vi "Binary Morphological Reconstruction.vi"() -> ()   [LabVIEW 2014]
doc: "This example demonstrates the use of binary morphological reconstruction in the particle analysis. The example allows you to keep the particles completely inside the ROI, completely outside the ROI or on the ROI."
uses:
  <vilib>/vision/NI_Vision_Development_Module.lvlib
panel:
  in  "Operation":T1(ring)
  out "Reconstructed Image":T2(plugin-control)
  out "Image":T2(plugin-control)
  in  "Stop":bool
  # "Overview: Demonstrate the use of the Binary Morphology Reconstruction feature of Vision Development Module.\nRequirements: Vision Development Module.\nInstructions:\n1. Run the VI.\n2. Select the ROI in which you want to filter the objects. Press the <Ctrl> key to select multiple ROIs. \n3. Choose the required \"Operation\".\n  - Inner particles: Keeps all the particles completely inside the ROI.\n  - Outer particles: Keeps the particles completely outside the ROI.\n  - Boundary particles: Keeps the particles which are touching the boundary."
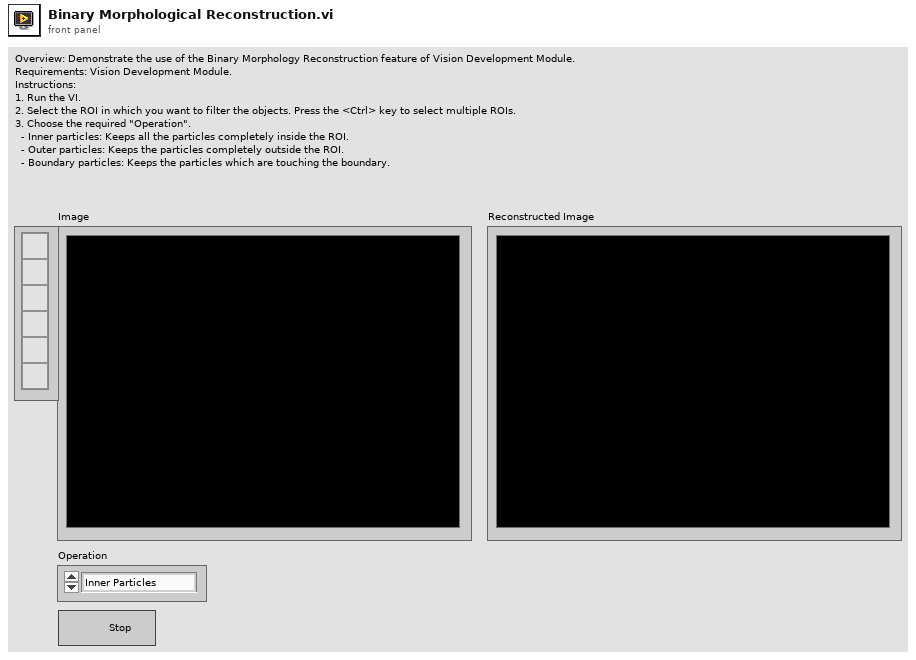
[diagram p1: front panel]
types:
  T1 = enum16{"Inner Particles", "Outer Particles", "Boundary Particles"}
  T2 = typedef "IMAQ Image.ctl" = refnum<image>
  T3 = typedef "Image Type" = u32
  T4 = cluster{"Global Rectangle":i32[], "Contours":cluster{"Contour Type":u32, "ROI Type":u32, "Points":i32[]}[]}
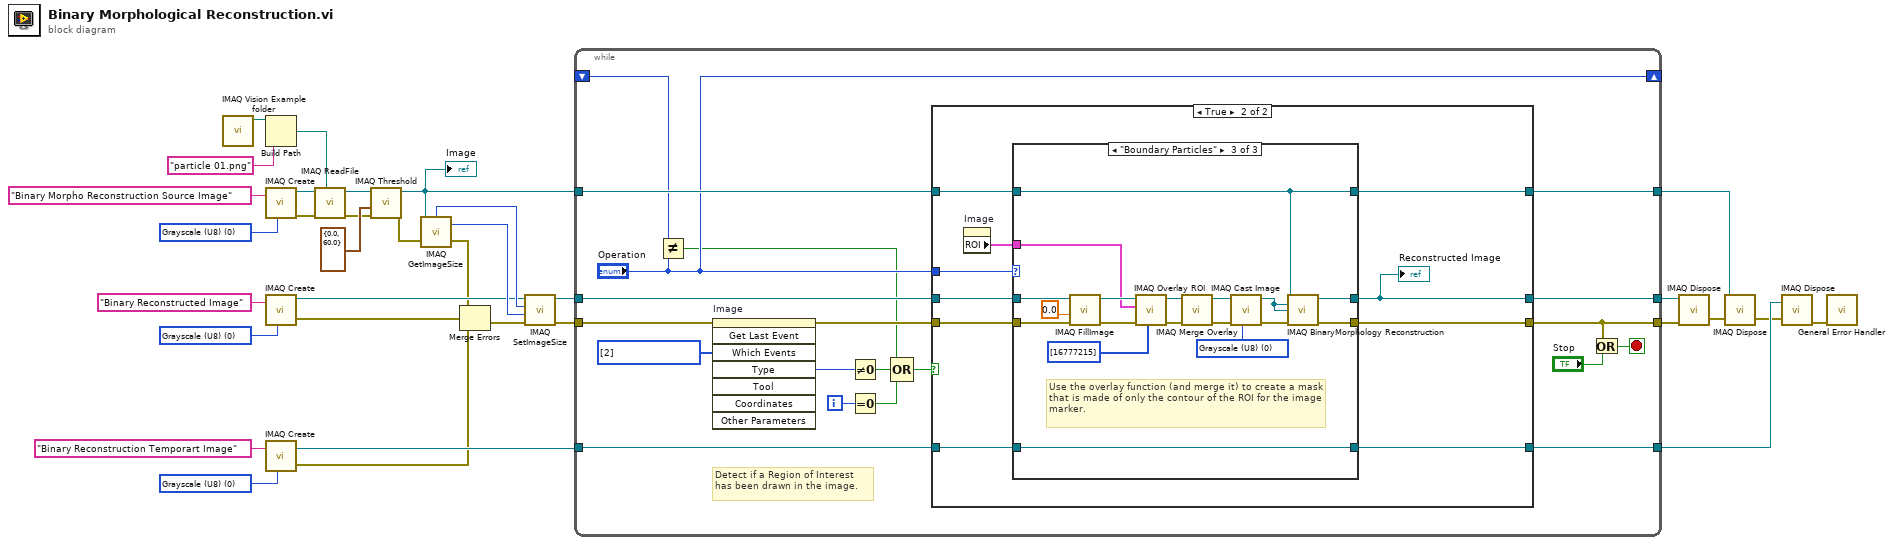
[diagram p0: block diagram]
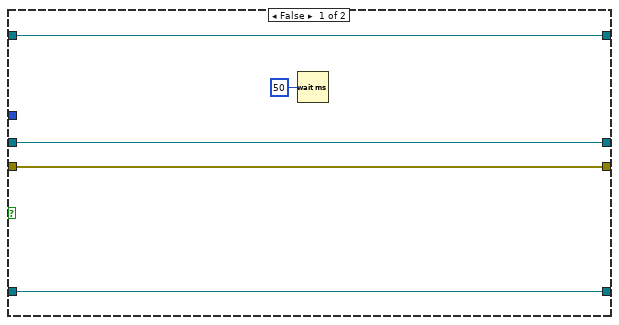
[diagram p2: hidden frame]
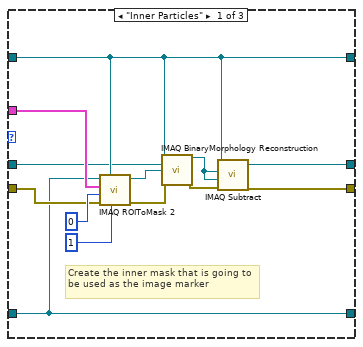
[diagram p3: hidden frame]
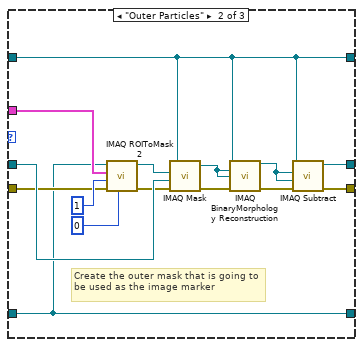
[diagram p4: hidden frame]
diagram:
  w23 = T3 0 items=["Grayscale (U8)", "Grayscale (I16)", "Grayscale (SGL)", "Complex (CSG)", "RGB (U32)", "HSL (U32)", "RGB (U64)", "Grayscale (U16)"] ("Image Type")
  w25 = T3 0 items=["Grayscale (U8)", "Grayscale (I16)", "Grayscale (SGL)", "Complex (CSG)", "RGB (U32)", "HSL (U32)", "RGB (U64)", "Grayscale (U16)"] ("Image Type")
  w26 = T3 0 items=["Grayscale (U8)", "Grayscale (I16)", "Grayscale (SGL)", "Complex (CSG)", "RGB (U32)", "HSL (U32)", "RGB (U64)", "Grayscale (U16)"] ("Image Type")
  n1 = call "IMAQ Vision Example folder.vi"() -> ("Example Image Path"=w32:path)  [unwired: 11 in]
  n2 = Build Path(base path=w32, name or relative path="particle 01.png") -> (appended path=w1:path)
  n3 = call "IMAQ Create"("Image Name"="Binary Morpho Reconstruction Source Image", "Image Type"=w25) -> ("New Image"=w29:T2, "error out"=w14:errorcluster)  [unwired: 2 in, 1 out]
  n4 = call "IMAQ Create"("Image Name"="Binary Reconstructed Image", "Image Type"=w26) -> ("New Image"=w19:T2, "error out"=w11:errorcluster)  [unwired: 2 in, 1 out]
  n5 = call "IMAQ Create"("Image Name"="Binary Reconstruction Temporart Image", "Image Type"=w23) -> ("New Image"=w20:T2, "error out"=w10:errorcluster)  [unwired: 2 in, 1 out]
  n6 = call "IMAQ ReadFile"("File Path"=w1, "error in (no error)"=w14, "Image"=w29) -> ("error out"=w13:errorcluster, "Image Out"=w17:T2)  [unwired: 2 in, 5 out]
  n7 = call "IMAQ Threshold"("error in (no error)"=w13, "Range"=cluster{"Lower value":sgl, "Upper value":sgl} {"Lower value"=0.0, "Upper value"=60.0}, "Image Src"=w17) -> ("error out"=w12:errorcluster, "Image Dst Out"=w15:T2)  [unwired: 3 in, 4 out]
  "Image" <- w15
  n8 = call "IMAQ GetImageSize"("Image"=w15, "error in (no error)"=w12) -> ("Y Resolution"=w21:i32, "X Resolution"=w22:i32, "error out"=w7:errorcluster)  [unwired: 2 out]
  n9 = Merge Errors(w7, w11, w10) -> (w9:errorcluster)
  n10 = call "IMAQ SetImageSize"("error in (no error)"=w9, "Y Resolution"=w21, "X Resolution"=w22, "Image"=w19) -> ("error out"=w8:errorcluster, "Image Out"=w18:T2)  [unwired: 1 out]
  n11 = while {
    tunnel: w15 -> [w53]
    tunnel: w18 -> [w52]
    tunnel: [w51] -> w28
    tunnel: [w50] -> w27
    tunnel: w20 -> [w49]
    shift-right: ["Operation"] -> _
    shift-left: _ -> [w48]
    tunnel: w8 -> [w44]
    tunnel: [w36] -> w5
    tunnel: [w42] -> w6
    i -> [w39]
    stop <- w34 stop-if-true
    w45 = i32[] [2] items=["No Event"=0, "Click Event"=1, "Draw Event"=2, "Size Event"=4, "Scroll Event"=5, "Double Click Event"=8] ("Which Events")
    # "Detect if a Region of Interest has been drawn in the image."
    n12 = Not Equal?(x=w48, y="Operation") -> (x != y?=w41:bool)
    n13 = invoke on="Image" class="ImageControl" method="Get Last Event"(error in=w44, "Which Events"=w45) -> (error out=w43:errorcluster, "Type"=w46:i32)  [unwired: 6 in, 6 out]
    n14 = Not Equal To 0?(x=w46) -> (x != 0?=w40:bool)
    n15 = Equal To 0?(x=w39) -> (x = 0?=w38:bool)
    n16 = Compound Arithmetic op=OR(w41, w40, w38) -> (w37:bool)
    n17 = case shown="True" w37 {
      tunnel: w53 -> [w58 w68]
      tunnel: w52 -> [w57 w67]
      tunnel: [w57 w66] -> w51
      tunnel: [w58 w65] -> w50
      tunnel: w49 -> [w55 w60]
      tunnel: "Operation" -> [_ w63]
      tunnel: w43 -> [w56 w62]
      tunnel: [w56 w61] -> w36
      tunnel: [w55 w59] -> w42
      frame False {
        n18 = Wait (ms)(milliseconds to wait=u32 50) -> ()  [unwired: 1 out]
      }
      frame True {
        n19 = property on="Image" class="ImageControl"() -> ("ROI"=w64:T4)  [unwired: 2 in, 2 out]
        n20 = case shown="\"Boundary Particles\"" w63 {
          tunnel: w68 -> [w76 w88 w111]
          tunnel: w67 -> [w74 w89 w103]
          tunnel: w60 -> [w69 w82 w112]
          tunnel: [w78 w91 w114] -> w66
          tunnel: w64 -> [w77 w90 w104]
          tunnel: [w76 w88 w111] -> w65
          tunnel: w62 -> [w73 w87 w102]
          tunnel: [w70 w83 w113] -> w61
          tunnel: [w69 w82 w112] -> w59
          frame "Inner Particles" {
            # "Create the inner mask that is going to be used as the image marker"
            n21 = call "IMAQ ROIToMask 2"("Background Value (0)"=1, "Image Model"=w76, "error in (no error)"=w73, "Filling Value (255)"=0, "ROI Descriptor"=w77, "Image"=w69) -> ("error out"=w72:errorcluster, "Image Out"=w75:T2)  [unwired: 4 out]
            n22 = call "IMAQ BinaryMorphology Reconstruction"("Image Src"=w76, "Image Dst"=w74, "Image Marker"=w75, "error in (no error)"=w72) -> ("Image Dst Out"=w79:T2, "error out"=w71:errorcluster)  [unwired: 4 in, 6 out]
            n23 = call "IMAQ Subtract"("Image Src A"=w76, "Image Dst"=w79, "Image Src B"=w79, "error in (no error)"=w71) -> ("Image Dst Out"=w78:T2, "error out"=w70:errorcluster)  [unwired: 1 in, 2 out]
          }
          frame "Outer Particles" {
            # "Create the outer mask that is going to be used as the image marker"
            n24 = call "IMAQ ROIToMask 2"("Background Value (0)"=0, "error in (no error)"=w87, "Filling Value (255)"=1, "ROI Descriptor"=w90, "Image"=w82) -> ("error out"=w86:errorcluster, "Image Out"=w94:T2)  [unwired: 1 in, 4 out]
            n25 = call "IMAQ Mask"("error in (no error)"=w86, "Image Dst"=w89, "Image Mask"=w94, "Image Src"=w88) -> ("error out"=w85:errorcluster, "Image Dst Out"=w93:T2)  [unwired: 1 out]
            n26 = call "IMAQ BinaryMorphology Reconstruction"("Image Src"=w88, "Image Dst"=w93, "Image Marker"=w93, "error in (no error)"=w85) -> ("Image Dst Out"=w92:T2, "error out"=w84:errorcluster)  [unwired: 4 in, 6 out]
            n27 = call "IMAQ Subtract"("Image Src A"=w88, "Image Dst"=w92, "Image Src B"=w92, "error in (no error)"=w84) -> ("Image Dst Out"=w91:T2, "error out"=w83:errorcluster)  [unwired: 1 in, 2 out]
          }
          frame "Boundary Particles" {
            w106 = T3 0 items=["Grayscale (U8)", "Grayscale (I16)", "Grayscale (SGL)", "Complex (CSG)", "RGB (U32)", "HSL (U32)", "RGB (U64)", "Grayscale (U16)"] ("Image Type")
            # "Use the overlay function (and merge it) to create a mask that is made of only the contour of the ROI for the image marker."
            n28 = call "IMAQ FillImage"("error in (no error)"=w102, "Pixel Value (U8, U16, I16, Float)"=sgl 0.0, "Image"=w103) -> ("error out"=w101:errorcluster, "Image Out"=w109:T2)  [unwired: 4 in, 3 out]
            n29 = call "IMAQ Overlay ROI"("Colors (Green)"=u32[] [16777215], "error in (no error)"=w101, "ROI Descriptor"=w104, "Image"=w109) -> ("error out"=w100:errorcluster, "Image Out"=w110:T2)  [unwired: 2 in, 4 out]
            n30 = call "IMAQ Merge Overlay"("error in (no error)"=w100, "Image Src"=w110) -> ("error out"=w99:errorcluster, "Image Dst Out"=w107:T2)  [unwired: 3 in, 5 out]
            n31 = call "IMAQ Cast Image"("Image Type"=w106, "error in (no error)"=w99, "Image Src"=w107) -> ("error out"=w98:errorcluster, "Image Dst Out"=w97:T2)  [unwired: 3 in, 4 out]
            n32 = call "IMAQ BinaryMorphology Reconstruction"("Image Src"=w111, "Image Dst"=w97, "Image Marker"=w97, "error in (no error)"=w98) -> ("Image Dst Out"=w114:T2, "error out"=w113:errorcluster)  [unwired: 4 in, 6 out]
          }
        }
        "Reconstructed Image" <- w66
      }
    }
    n33 = Or(x=w36, y="Stop") -> (x .or. y?=w34:bool)
  }
  n34 = call "IMAQ Dispose"("Image"=w28, "error in (no error)"=w5) -> ("error out"=w4:errorcluster)  [unwired: 1 in, 3 out]
  n35 = call "IMAQ Dispose"("Image"=w27, "error in (no error)"=w4) -> ("error out"=w3:errorcluster)  [unwired: 1 in, 3 out]
  n36 = call "IMAQ Dispose"("Image"=w6, "error in (no error)"=w3) -> ("error out"=w2:errorcluster)  [unwired: 1 in, 3 out]
  n37 = call <vilib>:"General Error Handler.vi"("error in (no error)"=w2) -> ()  [unwired: 10 in, 5 out]
